vi "Generic command handler.vi"(8 "error in (no error)":errorcluster, 10 "Message in":refnum<class "GenericMessage.lvclass">, 11 "Retiga in":refnum<class "Retiga.lvclass">) -> (0 "error out":errorcluster, 2 "value":string, 3 "Retiga out":refnum<class "Retiga.lvclass">)   [LabVIEW 2012, in "Retiga.lvclass"]
doc: "The generic_command_handler processes the command 'generic'. Commands which are not part of the predefined list of commands fall under the 'generic' command for special activity."
uses:
  Retiga.lvclass
  <vilib>/Distrio/Murmex/GenericMessage/GenericMessage.lvclass
  <vilib>/Distrio/Murmex/Murmex/Murmex.lvclass
  Retiga.lvclass/Retiga.ctl
  <vilib>/Distrio/Murmex/ProceedMessage/ProceedMessage.lvclass
panel:
  out "elapsed time (ms)":u32
  # "This method is called when the GENERIC\ntrigger is sent. \n\nOverride this method when your component needs to\nrespond to this trigger. \n\nCall parent for proper implementation"
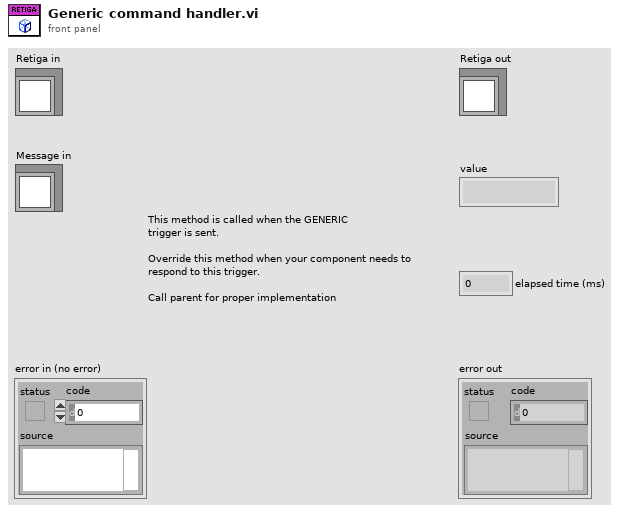
[diagram p1: front panel]
types:
  T1 = typedef "IMAQ Image.ctl" = refnum<image>
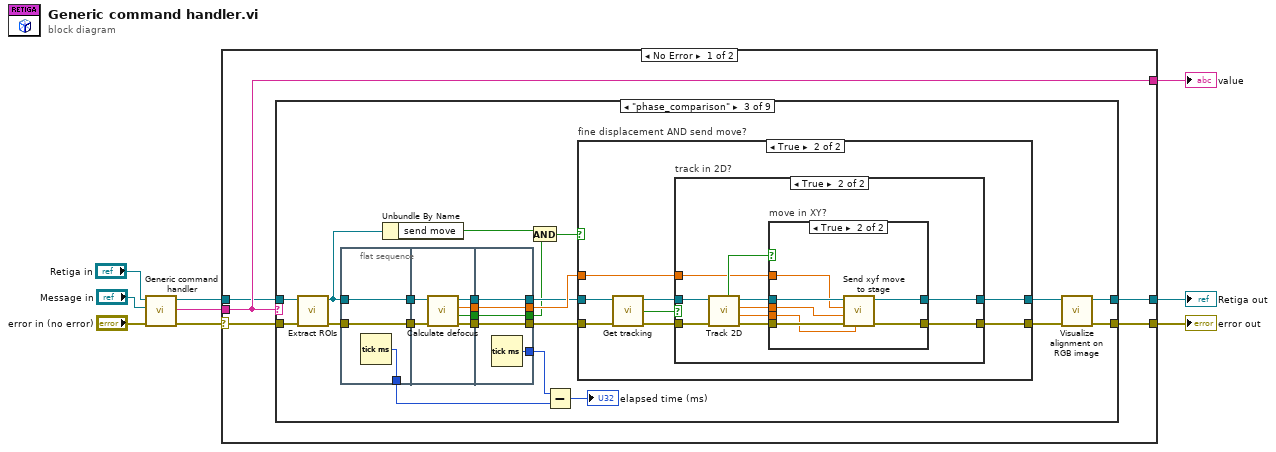
[diagram p0: block diagram]
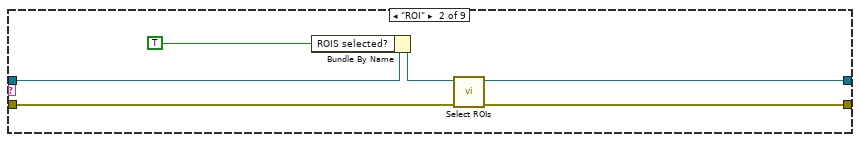
[diagram p3: hidden frame]
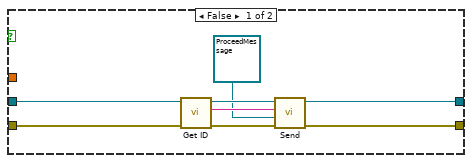
[diagram p4: hidden frame]
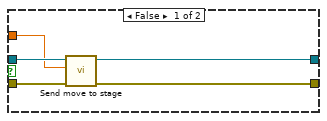
[diagram p5: hidden frame]
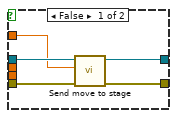
[diagram p6: hidden frame]
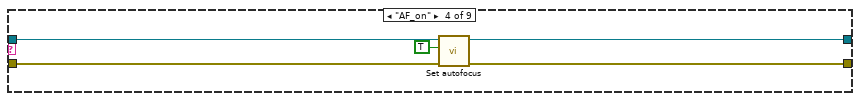
[diagram p7: hidden frame]
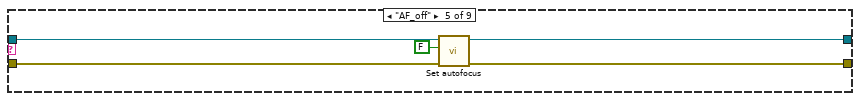
[diagram p8: hidden frame]
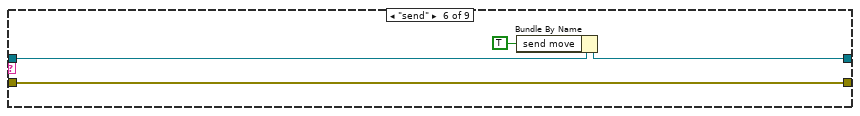
[diagram p9: hidden frame]
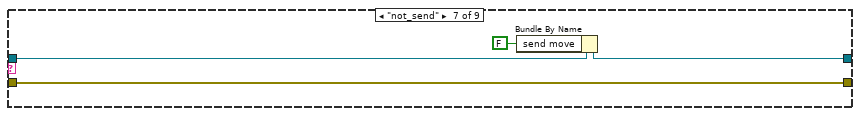
[diagram p10: hidden frame]
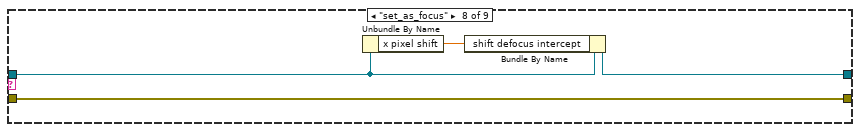
[diagram p11: hidden frame]
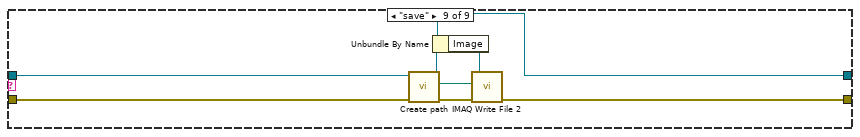
[diagram p12: hidden frame]
diagram:
  n1 = call-parent "Generic command handler.vi"("error in (no error)"="error in (no error)", "Message in"="Message in", "Murmex in"="Retiga in") -> ("error out"=w6:errorcluster, "value"=w4:string, "Murmex out"=w5:refnum<class "Retiga.lvclass">)  [unwired: 6 in]
  n2 = case shown="No Error" w6 {
    selector: w6 -> [w12 w133]
    tunnel: w5 -> [w10 w134]
    tunnel: w4 -> [w14 w132]
    tunnel: [w11 w134] -> w3
    tunnel: [w13 w133] -> w2
    tunnel: [w14 w132] -> w1
    frame No Error {
      n3 = case shown="\"phase_comparison\"" w14 {
        tunnel: [w16 w18 w38 w104 w109 w114 w118 w121 w126] -> w13
        tunnel: w12 -> [w16 w19 w44 w107 w112 w114 w118 w121 w130]
        tunnel: [w15 w17 w36 w105 w110 w115 w119 w122 w125] -> w11
        tunnel: w10 -> [w15 w22 w45 w106 w111 w116 w120 w124 w131]
        frame Default {
        }
        frame "ROI" {
          n4 = Bundle By Name(cluster=w22, "ROIS selected?"=TRUE ("runtime.ROIS selected?")) -> (w20:refnum<class "Retiga.lvclass">)
          n5 = call-dynamic "Select ROIs.vi"("error in (no error)"=w19, "Retiga in"=w20) -> ("error out"=w18:errorcluster, "Retiga out"=w17:refnum<class "Retiga.lvclass">)  [unwired: 8 in]
        }
        frame "phase_comparison" {
          n6 = call-dynamic "Extract ROIs.vi"("error in (no error)"=w44, "Retiga in"=w45) -> ("error out"=w43:errorcluster, "Retiga out"=w35:refnum<class "Retiga.lvclass">)  [unwired: 8 in]
          n7 = flat-sequence {
            tunnel: w35 -> [w47]
            tunnel: w43 -> [w48]
            tunnel: [w48] -> w27
            tunnel: [w47] -> w26
            tunnel: [w46] -> w24
            tunnel: [w53] -> w31
            tunnel: [w52] -> w30
            tunnel: [w51] -> w29
            tunnel: [w49] -> w28
            tunnel: w27 -> [w54]
            tunnel: w26 -> [w50]
            tunnel: [w56] -> w33
            tunnel: [w57] -> w40
            tunnel: [w58] -> w41
            tunnel: [w59] -> w42
            tunnel: w31 -> [w59]
            tunnel: w30 -> [w58]
            tunnel: w29 -> [w57]
            tunnel: w28 -> [w56]
            tunnel: [w55] -> w25
            frame #0 {
              n8 = Tick Count (ms)() -> (millisecond timer value=w46:u32)
            }
            frame #1 {
              n9 = call-dynamic "Calculate defocus.vi"("error in (no error)"=w54, "Retiga in"=w50) -> ("error out"=w52:errorcluster, "fine?"=w49:bool, "translation out"=w53:dbl[unit], "Retiga out"=w51:refnum<class "Retiga.lvclass">)  [unwired: 6 in]
            }
            frame #2 {
              n10 = Tick Count (ms)() -> (millisecond timer value=w55:u32)
            }
          }
          n11 = Unbundle By Name(w35) -> ("send move"=w34:bool)
          n12 = And(x=w34, y=w33) -> (x .and. y?=w32:bool)
          n13 = Subtract(x=w25, y=w24) -> (x-y=→"elapsed time (ms)":u32)
          n14 = case "fine displacement AND send move?" shown="True" w32 {
            tunnel: w42 -> [_ w73]
            tunnel: w41 -> [w65 w70]
            tunnel: w40 -> [w63 w72]
            tunnel: [w66 w75] -> w37
            tunnel: [w67 w74] -> w39
            frame False {
              n15 = call <vilib>:"Get ID.vi"("error in (no error)"=w65, "Murmex in"=w63) -> ("error out"=w64:errorcluster, "component id"=w61:string, "Murmex out"=w62:refnum<class "Retiga.lvclass">)  [unwired: 7 in]
              n16 = call <vilib>:"Send.vi"("error in (no error)"=w64, "Message"=refnum<class "ProceedMessage.lvclass"> refnum ("Distrio Murmex 1.5:ProceedMessage"), "recipient"=w61, "Murmex in"=w62) -> ("error out"=w67:errorcluster, "Murmex out"=w66:refnum<class "Retiga.lvclass">)  [unwired: 6 in]
            }
            frame True {
              n17 = call-dynamic "Get tracking.vi"("error in (no error)"=w70, "Retiga in"=w72) -> ("error out"=w69:errorcluster, "2D tracking?"=w68:bool, "Retiga out"=w71:refnum<class "Retiga.lvclass">)  [unwired: 7 in]
              n18 = case "track in 2D?" shown="True" w68 {
                tunnel: [w80 w84] -> w75
                tunnel: [w79 w85] -> w74
                tunnel: w69 -> [w78 w89]
                tunnel: w71 -> [w77 w90]
                tunnel: w73 -> [w76 w81]
                frame False {
                  n19 = call-dynamic "Send move to stage.vi"("error in (no error)"=w78, "move to send"=w76, "Retiga in"=w77) -> ("error out"=w79:errorcluster, "Retiga out"=w80:refnum<class "Retiga.lvclass">)  [unwired: 7 in]
                }
                frame True {
                  n20 = call-dynamic "Track 2D.vi"("error in (no error)"=w89, "Retiga in"=w90) -> ("error out"=w87:errorcluster, "Y move"=w82:sgl[unit], "X move"=w83:sgl[unit], "Retiga out"=w86:refnum<class "Retiga.lvclass">, "move in XY?"=w88:bool)  [unwired: 5 in]
                  n21 = case "move in XY?" shown="True" w88 {
                    tunnel: w87 -> [w94 w101]
                    tunnel: w86 -> [w95 w102]
                    tunnel: [w91 w100] -> w85
                    tunnel: [w92 w99] -> w84
                    tunnel: w83 -> [_ w98]
                    tunnel: w82 -> [_ w97]
                    tunnel: w81 -> [w93 w96]
                    frame False {
                      n22 = call-dynamic "Send move to stage.vi"("error in (no error)"=w94, "move to send"=w93, "Retiga in"=w95) -> ("error out"=w91:errorcluster, "Retiga out"=w92:refnum<class "Retiga.lvclass">)  [unwired: 7 in]
                    }
                    frame True {
                      n23 = call-dynamic "Send xyf move to stage.vi"("Y move to send"=w97, "error in (no error)"=w101, "X move to send"=w98, "focus move to send"=w96, "Retiga in"=w102) -> ("error out"=w100:errorcluster, "Retiga out"=w99:refnum<class "Retiga.lvclass">)  [unwired: 5 in]
                    }
                  }
                }
              }
            }
          }
          n24 = call-dynamic "Visualize alignment on RGB image.vi"("error in (no error)"=w39, "Retiga in"=w37) -> ("error out"=w38:errorcluster, "Retiga out"=w36:refnum<class "Retiga.lvclass">)  [unwired: 8 in]
        }
        frame "AF_on" {
          n25 = call-dynamic "Set autofocus.vi"("error in (no error)"=w107, "autofocusing?"=TRUE, "Retiga in"=w106) -> ("error out"=w104:errorcluster, "Retiga out"=w105:refnum<class "Retiga.lvclass">)  [unwired: 7 in]
        }
        frame "AF_off" {
          n26 = call-dynamic "Set autofocus.vi"("error in (no error)"=w112, "autofocusing?"=FALSE, "Retiga in"=w111) -> ("error out"=w109:errorcluster, "Retiga out"=w110:refnum<class "Retiga.lvclass">)  [unwired: 7 in]
        }
        frame "send" {
          n27 = Bundle By Name(cluster=w116, "send move"=TRUE ("runtime.cross correlation.send move")) -> (w115:refnum<class "Retiga.lvclass">)
        }
        frame "not_send" {
          n28 = Bundle By Name(cluster=w120, "send move"=FALSE ("runtime.cross correlation.send move")) -> (w119:refnum<class "Retiga.lvclass">)
        }
        frame "set_as_focus" {
          n29 = Unbundle By Name(w124) -> ("x pixel shift"=w123:dbl)
          n30 = Bundle By Name(cluster=w124, "shift defocus intercept"=w123) -> (w122:refnum<class "Retiga.lvclass">)
        }
        frame "save" {
          n31 = call-dynamic "Create path.vi"("error in (no error)"=w130, "Retiga in"=w131) -> ("error out"=w127:errorcluster, "full path"=w128:path, "Retiga out"=w125:refnum<class "Retiga.lvclass">)  [unwired: 7 in]
          n32 = Unbundle By Name(w125) -> ("Image"=w129:T1)
          n33 = call-poly "IMAQ Write File 2"("error in (no error)"=w127, "File Path"=w128, "Image"=w129) -> ("error out"=w126:errorcluster)  [unwired: 7 in, 1 out]
        }
      }
    }
    frame Error {
    }
  }
  "error out" <- w2
  "Retiga out" <- w3
  "value" <- w1
